vi "SE_HV200.SetVoltage.vi"(0 "i ref in":refnum<vi>, 2 "Set Voltage":dbl format="%.5f", 3 "Channel":i16, 4 "Time out":i32, 5 "error in (no error)":errorcluster) -> (14 "i ref out":refnum<vi>, 16 "timed out":bool, 19 "error out":errorcluster)   [LabVIEW 2014, in "SE_HV200.lvlib"]
doc: "Sets the Voltage at the Device. but first one should increase the current to set the voltage else the Voltage might not be set"
uses:
  SE_HV200.lvlib
  CSCore/CSSystem/CoreLib/CoreLib.lvlib
  CSCore/CSSystem/CoreDefs/CoreDefs.error_type.ctl
  CSlibraries-extern/DimLVEvent/LVDimInterface/LVDimInterface.lvlib
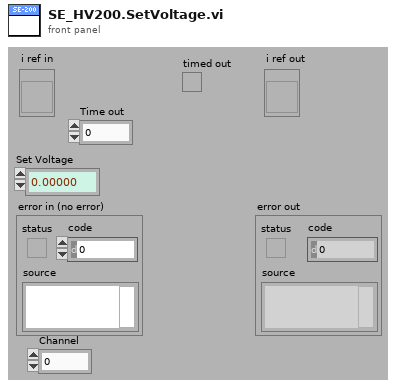
[diagram p1: front panel]
types:
  T1 = typedef "CoreDefs.error_type.ctl" = enum16{"no error", "can't load process", "can't unload process", "process does not exist", "can't install process", "can't remove process", "unknown function", "time out", "can't execute function", "duplicate queue name", "super not found", "caller queue invalid", "can't ping process", "unknown error", "VISA Error", "VISA timeout", "GPIB timeout", "GPIB error", "communication error", "data type mismatch", "can't read data from OPC server", "can't write data to OPC server", "OET error", "function not implemented", "process already exists", "invalid Shared Variable name", "error writing Shared Variable", "error reading Shared Variable", "invalid client name", "corrupt database", "unknown class", "call not authorized", "parameter out of range", "OET timeout: can't get data to modify", "invalid queue name", "requested operation incompatible with current state", "event undefined", "event disabled", "state undefined", "caller is not a friend", "EventBuilder: bad eventID", "EventBuilder: no DAQ devices", "a thread must not stop itself", "UNUSED ELEMENT4", "DiscArchiver: eventData incomplete", "DiscArchiver: eventData does not belong to run", "DiscArchiver: can't open file", "DiscArchiver: can't write to file", "DiscArchiver: available disc space low", "can't acquire semaphore", "error reading data from database", "notifier object is not existing", "can't register process", "can't unregister process", "illegal event type", "object disabled", "object already exists", "can't change state", "Instrument not found", "no connection to remote node", "invalid reference", "N/A", "UNUSED ELEMENT 1", "element not found", "illegal TCP/IP connection detected", "object does not exist", "invalid access ID", "unknown CS system", "invalid privilige", "unsupported data type", "unsupported server type", "IO server already exists", "Shared Variable already exists"}
  T2 = typedef "SE_HV200.lvlib/SE_HV200.i attribute.ctl" = cluster{"SetStatus":bool, "actVoltageID":i32, "VISA resource name in":refnum<visa-resource-name>, "Device name":string, "PSRange":i32, "nomVoltageID":i32, "actStatusID":i32, "NomVoltage":dbl[], "ActVoltage":dbl[], "DefaultChannel":i32}
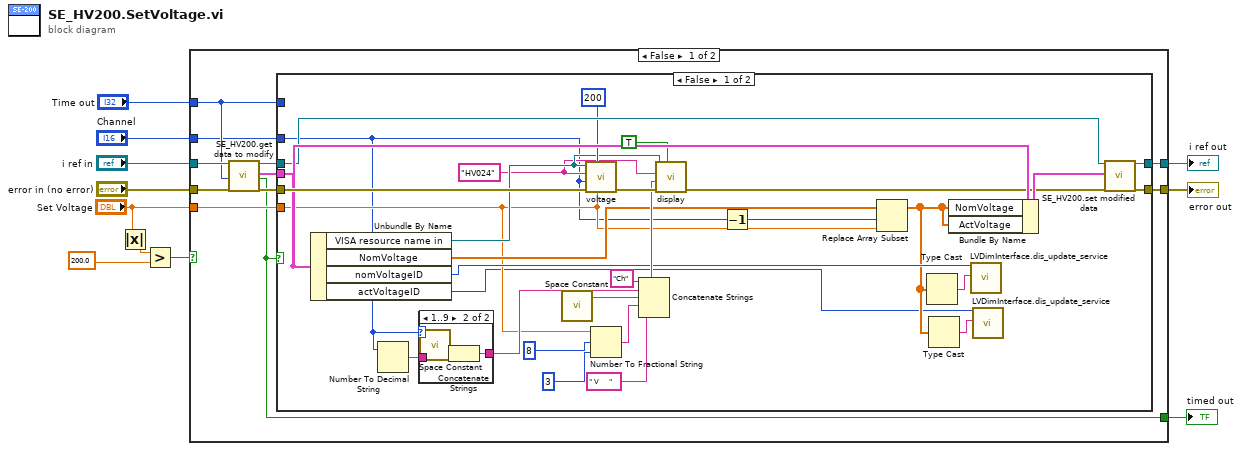
[diagram p0: block diagram]
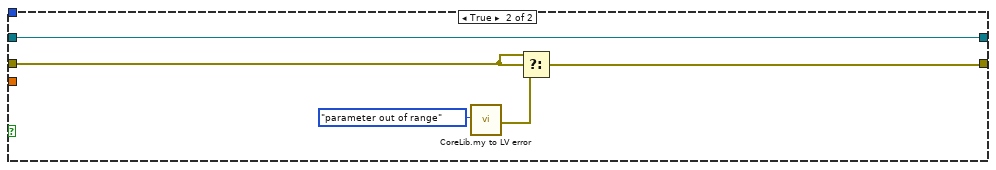
[diagram p4: hidden frame]
diagram:
  n1 = Absolute Value(x="Set Voltage") -> (abs(x)=w2:dbl)
  n2 = Greater?(x=w2, y=200.0) -> (0:w6:bool)
  n3 = case shown="False" w6 {
    tunnel: [w22 w59] -> w11
    tunnel: "Set Voltage" -> [w21 _]
    tunnel: [w20 w63] -> w10
    tunnel: "i ref in" -> [w18 w63]
    tunnel: "error in (no error)" -> [w16 w61]
    tunnel: "Time out" -> [w17 _]
    tunnel: [w13 _] -> w5
    tunnel: "Channel" -> [w12 _]
    frame False {
      n4 = call "SE_HV200.get data to modify.vi"("i ref in"=w18, "ms timeout (10000)"=w17, "error in (no error)"=w16) -> ("i ref out"=w19:refnum<vi>, "i attribute"=w14:T2, "timed out"=w13:bool, "error out"=w15:errorcluster)  [unwired: 13 in]
      n5 = case shown="False" w13 {
        tunnel: w14 -> [w49 _]
        tunnel: w15 -> [w50 w57]
        tunnel: [w51 w57] -> w22
        tunnel: w21 -> [w28 _]
        tunnel: w19 -> [w47 w58]
        tunnel: [w52 w58] -> w20
        tunnel: w17 -> [_ _]
        tunnel: w12 -> [w27 _]
        frame False {
          w34 = "HV024"
          n6 = Unbundle By Name(w49) -> ("VISA resource name in"=w35:refnum<visa-resource-name>, "NomVoltage"=w31:dbl[], "nomVoltageID"=w30:i32, "actVoltageID"=w23:i32)
          n7 = Number To Decimal String(number=w27) -> (decimal integer string=w33:string)  [unwired: 1 in]
          n8 = case shown="1..9" w27 {
            tunnel: w33 -> [w53 w56]
            tunnel: [w53 w54] -> w32
            frame Default {
            }
            frame 1..9 {
              n9 = call <vilib>:"Space Constant.vi"() -> ("String"=w55:string)
              n10 = Concatenate Strings(w55, w56) -> (w54:string)
            }
          }
          n11 = call <vilib>:"Space Constant.vi"() -> ("String"=w36:string)
          n12 = call "voltage.vi"("Voltage"=w28, "Span"=200, "Error in"=w50, "Channel nr."=w27, "Device name"=w34, "VISA resource name in"=w35) -> ("Error out"=w41:errorcluster)  [unwired: 3 in, 2 out]
          n13 = Number To Fractional String(number=w28, width (-)=8, precision (6)=3) -> (F-format string=w45:string)  [unwired: 1 in]
          n14 = Concatenate Strings("Ch" ("string"), w32, w36, w45, " V     " ("string")) -> (w39:string)
          n15 = call "display.vi"("Next free line"=TRUE, "Error in"=w41, "Display String"=w39, "Device name"=w34, "VISA resource name in"=w35) -> ("Error out"=w40:errorcluster)  [unwired: 5 in, 1 out]
          n16 = Decrement(x=w27) -> (x-1=w26:i16)
          n17 = Replace Array Subset(array=w31, new element=w28, index=w26) -> (w24:dbl[])
          n18 = Type Cast(x=w24) -> (*(type *) &x=w29:string)  [unwired: 1 in]
          n19 = Type Cast(x=w24) -> (*(type *) &x=w25:string)  [unwired: 1 in]
          n20 = Bundle By Name(cluster=w49, "NomVoltage"=w24, "ActVoltage"=w24) -> (w48:T2)
          n21 = call "LVDimInterface.dis_update_service.vi"("my_serviceID"=w30, "data"=w29) -> ()  [unwired: 15 in, 3 out]
          n22 = call "LVDimInterface.dis_update_service.vi"("my_serviceID"=w23, "data"=w25) -> ()  [unwired: 15 in, 3 out]
          n23 = call "SE_HV200.set modified data.vi"("i ref in"=w47, "i attribute"=w48, "error in (no error)"=w40) -> ("i ref out"=w52:refnum<vi>, "error out"=w51:errorcluster)  [unwired: 15 in]
        }
        frame True {
        }
      }
    }
    frame True {
      n24 = call "CoreLib.my to LV error.vi"("ErrorTypes"=CoreDefs.error_type."parameter out of range") -> ("myErrorCluster"=w60:errorcluster)  [unwired: 17 in, 1 out]
      n25 = Select(t=w61, s=w61, f=w60) -> (s? t:f=w59:errorcluster)
    }
  }
  "error out" <- w11
  "i ref out" <- w10
  "timed out" <- w5
